vi "USB5GetAi.vi"(7 "TimeOut":i32, 8 "错误输入（无错误）":errorcluster, 9 "Ai":sgl[][](array[numeric]), 10 "Points":u32, 11 "DevIndex":i32) -> (0 "错误输出":errorcluster, 1 "Ai Out":sgl[][](array[numeric]), 2 "AiFifoUsed":i32, 3 "DevIndex Out":i32)   [LabVIEW 2020]
uses:
  lib/x64/USB5000.dll
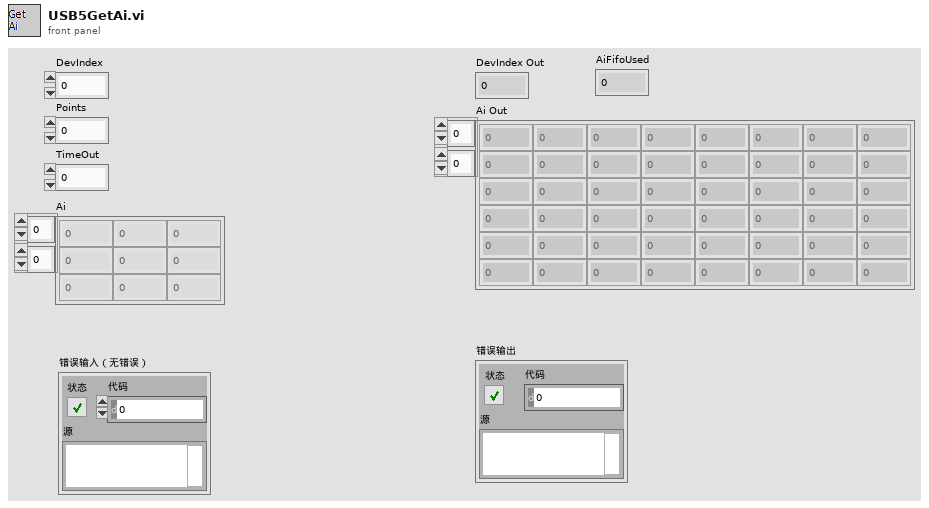
[diagram p1: front panel]
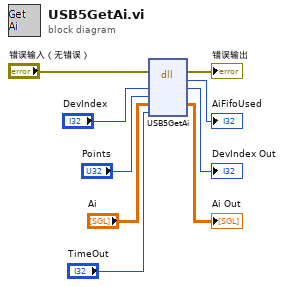
[diagram p0: block diagram]
diagram:
  n1 = dll-call lib="C:/Users/phosense/Downloads/USB-5000/usb5000_labview_cv/lib/x64/USB5000.dll" fn="USB5GetAi"(error in="错误输入（无错误）", "DevIndex"="DevIndex", "Points"="Points", "Ai"="Ai", "TimeOut"="TimeOut") -> (error out=→"错误输出":errorcluster, "返回类型"=→"AiFifoUsed":i32, "DevIndex"=→"DevIndex Out":i32, "Ai"=→"Ai Out":sgl[][])  [unwired: 4 in, 1 out]
